vi "Tracker File Reader.vi"() -> ()   [LabVIEW 2018]
uses:
  <vilib>/Utility/file.llb/Read Delimited Spreadsheet (string).vi
  <vilib>/Utility/file.llb/Write Delimited Spreadsheet (string).vi
panel:
  out "Output file path":path
  in  "Action 1":i32(ring) caption="Column to be saved" items=["X1_raw", "Y1_raw", "X2_raw", "Y2_raw", "Absolute_timestamp", "Relative_timestamp", "R", "phi", "alpha", "X", "Y", "w", "Current_zone", "Zones_preference", "TTL_inputs", "TTL_outputs", "Speed_mm_per_s", "Frame_OK"]
  in  "Action":i32(ring) caption="Required decimal devider" items=["No Change", "Comma", "Dot"]
  out "Input file path":path
  in  "Read the file:":bool
  in  "Save the column:":bool
  in  "DONE":bool
  out "error out":errorcluster
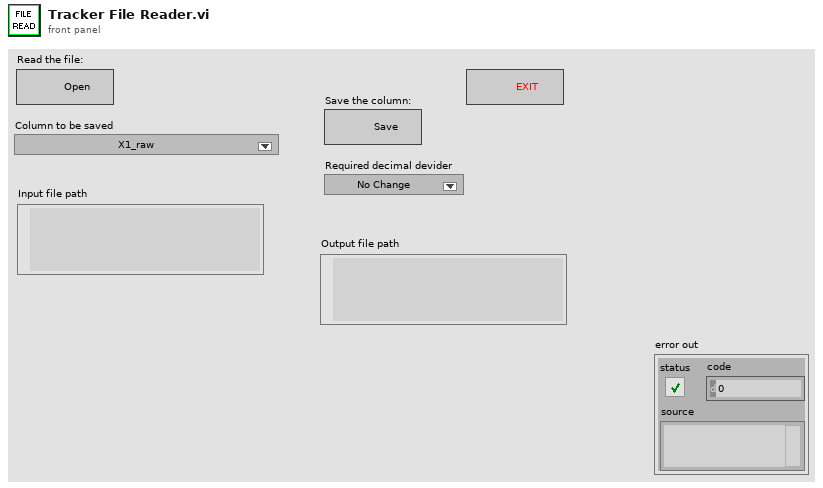
[diagram p1: front panel]
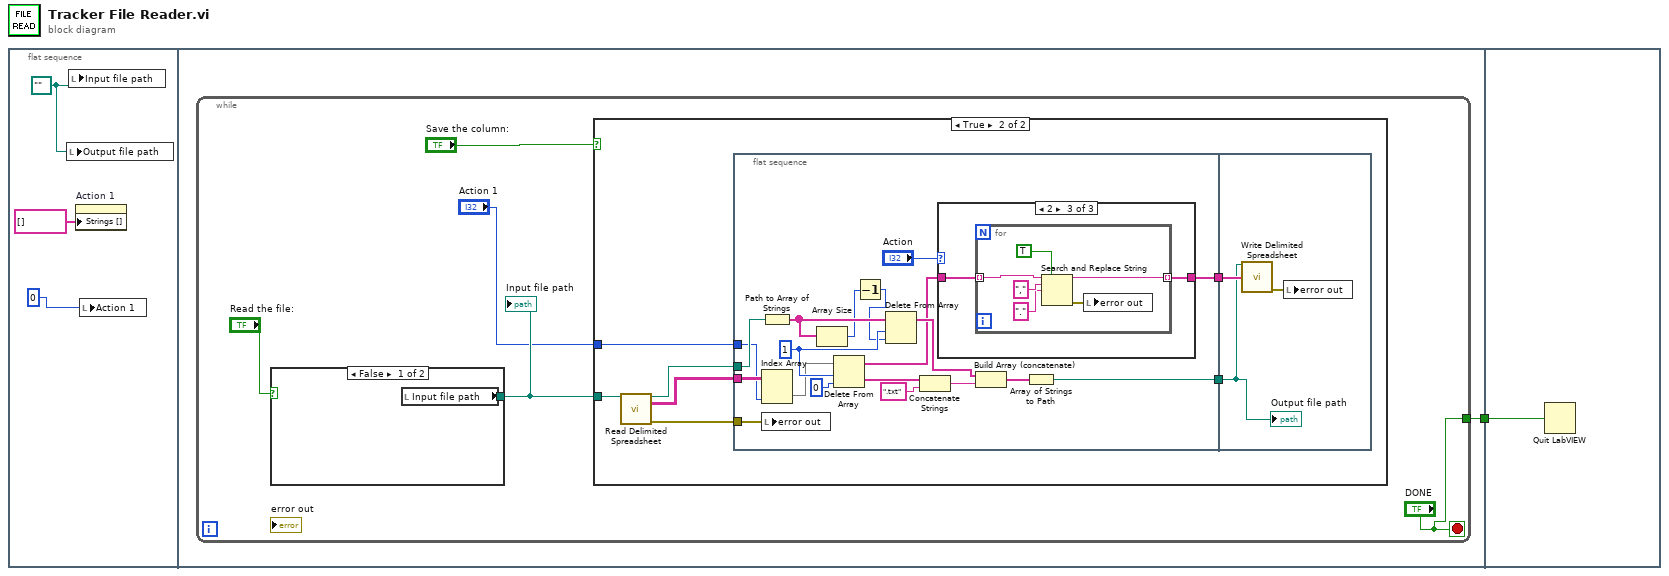
[diagram p0: block diagram]
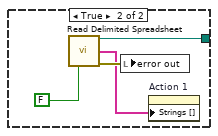
[diagram p2: hidden frame]
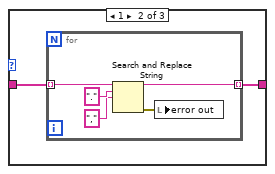
[diagram p5: hidden frame]
diagram:
  n1 = flat-sequence {
    tunnel: [w5] -> w1
    tunnel: w1 -> [w61]
    frame #0 {
      w3 = path "" ("new file path (Not A Path if cancelled)")
      n2 = local write "Output file path"(w3) -> ()
      n3 = local write "Input file path"(w3) -> ()
      n4 = property on="Action 1" class="Ring (strict)"("Strings []"=string[] []) -> ()  [unwired: 2 in, 2 out]
      n5 = local write "Action 1"(0 ("x-1")) -> ()
    }
    frame #1 {
      n6 = while {
        tunnel: ["DONE"] -> w5
        stop <- "DONE" stop-if-true
        n7 = case shown="False" "Read the file:" {
          tunnel: [w11 w14] -> w8
          frame False {
            n8 = local read "Input file path"() -> (w11:path)
          }
          frame True {
            n9 = call-poly <vilib>:"Read Delimited Spreadsheet.vi"("transpose? (F)"=FALSE ("append to file? (new file:F)")) -> ("new file path (Not A Path if cancelled)"=w14:path, "first row"=w12:string[], "error out"=w13:errorcluster)  [unwired: 9 in, 3 out]
            n10 = local write "error out"(w13) -> ()
            n11 = property on="Action 1" class="Ring (strict)"("Strings []"=w12) -> ()  [unwired: 2 in, 2 out]
          }
        }
        "Input file path" <- w8
        n12 = case shown="True" "Save the column:" {
          tunnel: "Action 1" -> [_ w20]
          tunnel: w8 -> [_ w22]
          frame False {
          }
          frame True {
            n13 = call-poly <vilib>:"Read Delimited Spreadsheet.vi"("file path (dialog if empty)"=w22) -> ("new file path (Not A Path if cancelled)"=w21:path, "all rows"=w16:string[][], "error out"=w19:errorcluster)  [unwired: 9 in, 3 out]
            n14 = flat-sequence {
              tunnel: w16 -> [w41]
              tunnel: w21 -> [w40]
              tunnel: w20 -> [w29]
              tunnel: w19 -> [w25]
              tunnel: [w31] -> w18
              tunnel: [w26] -> w17
              tunnel: w18 -> [w58]
              tunnel: w17 -> [w60]
              frame #0 {
                w38 = 1 ("length")
                n15 = Path to Array of Strings(0:w40) -> (2:w37:string[])  [unwired: 1 out]
                n16 = Index Array(array=w41, index (col)=w29) -> (element=w30:string[])  [unwired: 1 in]
                n17 = local write "error out"(w25) -> ()
                n18 = Array Size(array=w37) -> (size(s)=w24:i32)
                n19 = Delete From Array(array=w30, length=w38, index=0) -> (deleted portion=w36:string[], array with subset deleted=w27:string[])
                n20 = Decrement(x=w24) -> (x-1=w23:i32)
                n21 = Delete From Array(array=w37, length=w38, index=w23) -> (array with subset deleted=w34:string[])  [unwired: 1 out]
                n22 = Concatenate Strings(w36, ".txt" ("string")) -> (w33:string)
                n23 = case shown="2" "Action" {
                  tunnel: w27 -> [w42 w44 w51]
                  tunnel: [w42 w43 w50] -> w26
                  frame 0, Default {
                  }
                  frame 1 {
                    n24 = for {
                      tunnel: w44 -> [w49] mode=indexing
                      tunnel: [w45] -> w43 mode=indexing
                      n25 = Search and Replace String(input string=w49, search string=".", replace string="," ("replace string (\"\")")) -> (result string=w45:string, error out=w46:errorcluster)  [unwired: 5 in, 2 out]
                      n26 = local write "error out"(w46) -> ()
                    }
                  }
                  frame 2 {
                    n27 = for {
                      tunnel: w51 -> [w57] mode=indexing
                      tunnel: [w53] -> w50 mode=indexing
                      n28 = Search and Replace String(replace all?=TRUE ("replace all? (F)"), input string=w57, search string=",", replace string="." ("replace string (\"\")")) -> (result string=w53:string, error out=w54:errorcluster)  [unwired: 4 in, 2 out]
                      n29 = local write "error out"(w54) -> ()
                    }
                  }
                }
                n30 = Build Array (concatenate)(w34, w33) -> (w32:string[])
                n31 = Array of Strings to Path(0:w32) -> (2:w31:path)  [unwired: 1 in]
              }
              frame #1 {
                n32 = call-poly <vilib>:"Write Delimited Spreadsheet.vi"("file path (dialog if empty)"=w58, "1D data"=w60) -> ("error out"=w59:errorcluster)  [unwired: 12 in, 1 out]
                n33 = local write "error out"(w59) -> ()
                "Output file path" <- w58
              }
            }
          }
        }
      }
    }
    frame #2 {
      n34 = Quit LabVIEW(quit? (T)=w61) -> ()
    }
  }
